vi "Write.vi"(10 "Waveform Array":waveform(dbl)[](array[waveform]), 11 "Waveform Array in":refnum<class "Waveform Array.lvclass">) -> (3 "Waveform Array out":refnum<class "Waveform Array.lvclass">)   [LabVIEW 2020, in "Data.lvlib" / "Waveform Array.lvclass"]
doc: "Write Time Stamp Array."
uses:
  Waveform Array.lvclass
  Waveform Array.lvclass/Waveform Array.ctl
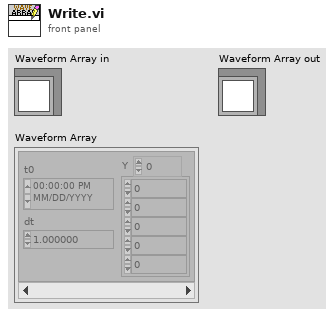
[diagram p1: front panel]
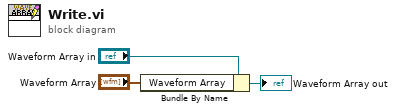
[diagram p0: block diagram]
diagram:
  n1 = Bundle By Name(cluster="Waveform Array in", "Waveform Array"="Waveform Array") -> (→"Waveform Array out":refnum<class "Waveform Array.lvclass">)
